vi "TDMS Main Page.vi"(8 "error in (no error)":errorcluster, 11 "Node Ptr":T2 format="%.0x") -> (0 "error out":errorcluster)   [LabVIEW 2011, in "TDMS Custom Device.lvlib"]
uses:
  TDMS Custom Device.lvlib
  <vilib>/NI Veristand/Custom Device API/Custom Device Item Ref.ctl
  <vilib>/NI Veristand/Custom Device API/Path Type.ctl
  <vilib>/NI Veristand/Custom Device API/Custom Device File Dependency.ctl
  <vilib>/NI Veristand/Custom Device API/Path Specification.ctl
  <vilib>/NI Veristand/Custom Device API/Custom Device Supported Target.ctl
  <vilib>/NI Veristand/Custom Device API/Set Item Property (Path).vi
  <vilib>/NI Veristand/Custom Device API/Custom Device API.lvlib
panel:
  out "# Samples":u32
  out "dt (sec)":dbl
  in  "Subheader":cluster{"Section Name":string}={"Section Name"="Buffering/Interpolation Default Settings"}
  in  "Fifo Depth":u32=200 min=1 max=400
  in  "Interpolation Width":i32=1 caption="The system uses this number of samples on either side of a point to be used by the above method. Increase to increase smoothness, decrease for performance." min=1 max=50
  in  "Interpolation Method":T1(ring)=enum."Linear"
  in  "View TDMS file":bool
  in  "Load Channels from File":bool
  in  "Header":cluster{"Section Name":string}={"Section Name"="TDMS Player Settings"}
  in  "Device Description (optional)":string
  in  "Name":string
  in  "Dependency":T4={"Source"={"TDMS Local Path"=path "", "Type"=enum."Absolute"}, "RT Path"=path "", "Force Download File?"=TRUE}
  # "Note: Used ONLY when 'Load Channels' is clicked."
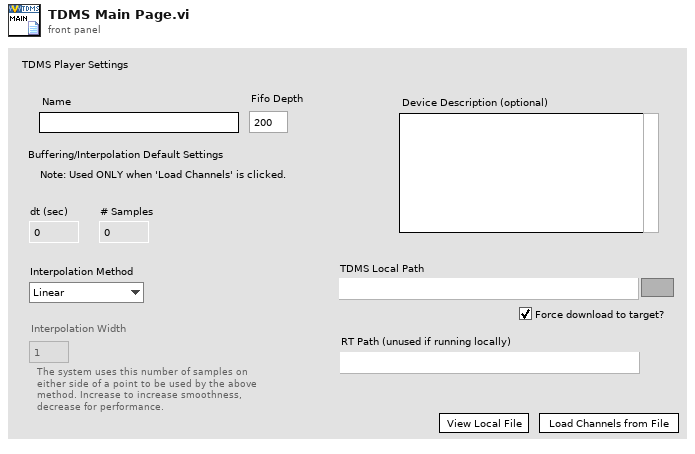
[diagram p1: front panel]
types:
  T1 = enum16{"Nearest", "Linear", "Spline", "Cubic Hermite", "Lagrange", "Polynomial"}
  T2 = typedef "Custom Device API.lvlib/Custom Device Item Ref.ctl" = u64
  T3 = typedef "Custom Device API.lvlib/Path Type.ctl" = enum16{"Absolute", "To Base", "To Common Data Dir", "To Application Data Dir"}
  T4 = cluster{"Source":cluster{"TDMS Local Path":path, "Type":T3}, "RT Path":path, "Force Download File?":bool}
  T5 = typedef "Custom Device API.lvlib/Custom Device Item Info.ctl" = cluster{"Name":string, "Is Channel":bool, "GUID":string}
  T6 = typedef "Custom Device API.lvlib/Custom Device File Dependency.ctl" = cluster{"Source":T7, "RT Destination":path, "ForceDownload?":bool, "SupportedTarget":T8, "Version":string}
  T7 = typedef "Custom Device API.lvlib/Path Specification.ctl" = cluster{"Path":path, "Type":T3}
  T8 = typedef "Custom Device API.lvlib/Custom Device Supported Target.ctl" = enum16{"All", "PharLap", "VxWorks", "Windows", "PharLap & Windows", "PharLap & VxWorks", "VxWorks & Windows"}
  T9 = typedef "Custom Device API.lvlib/Custom Device Channel.ctl" = cluster{"Type":T10, "Units":string, "Default Value":dbl, "Faultable":bool, "Scalable":bool}
  T10 = typedef "Custom Device API.lvlib/Custom Device Channel Type.ctl" = enum16{"Input", "Output"}
  T11 = enum8{"Enabled", "Disabled", "Disabled and Grayed Out"}
  T12 = typedef "Custom Device API.lvlib/Custom Device Commands.ctl" = enum16{"Default", "Item renamed", "Shutdown", "Dynamic button pressed"}
  T13 = cluster{bool, "dt (sec)":dbl, "Interpolation Method ":enum16{"Nearest", "Linear", "Spline", "Cubic Hermite", "Lagrange", "Polynomial"}, "Interpolation Width":i32}
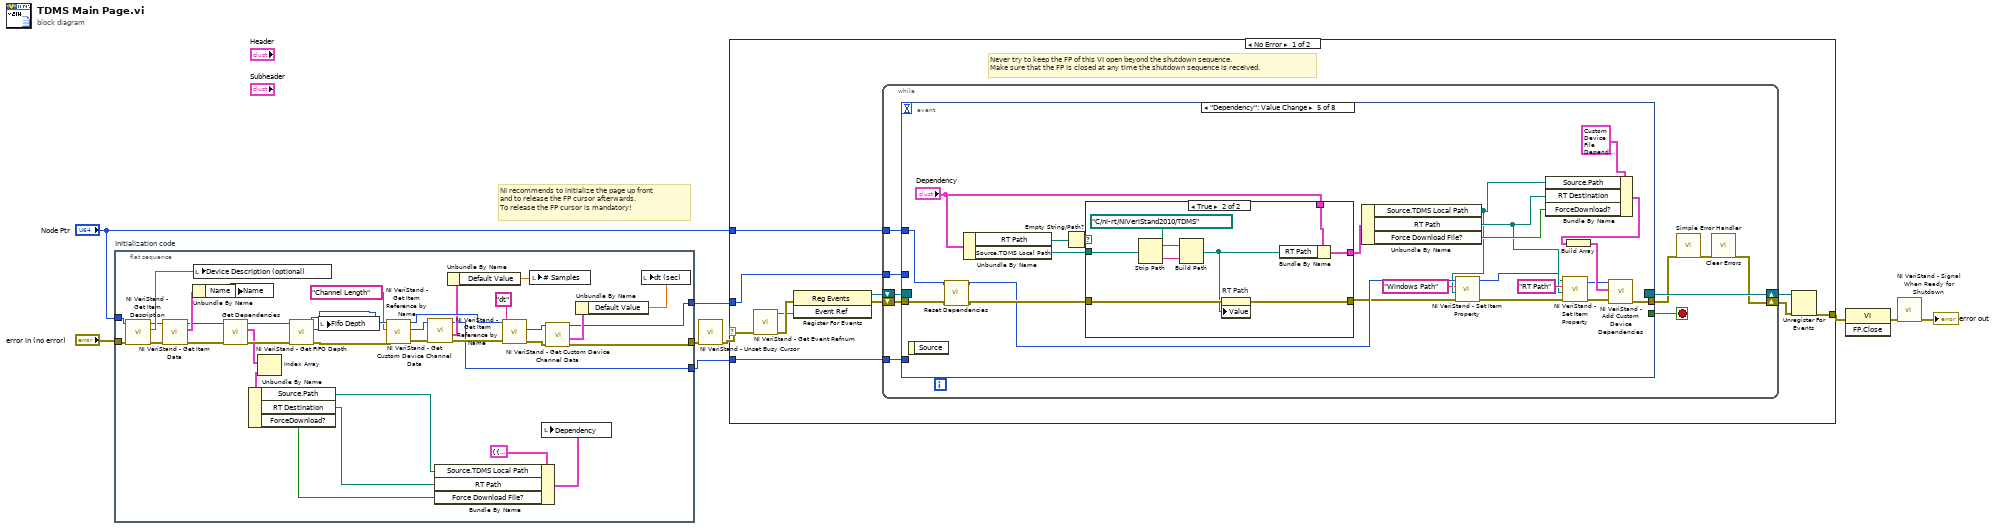
[diagram p0: block diagram]
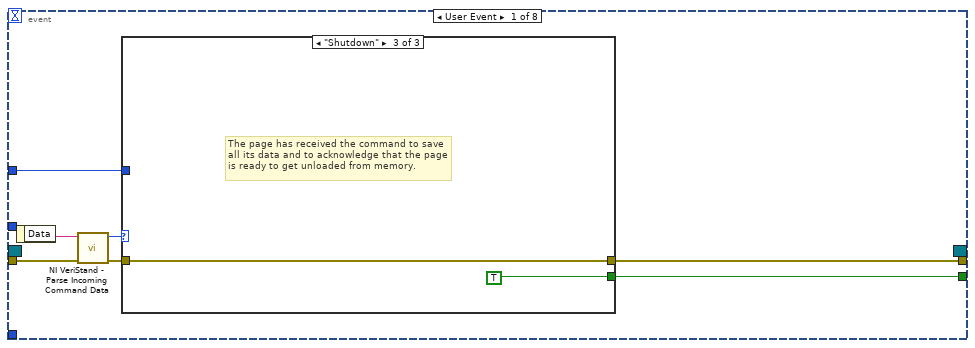
[diagram p2: hidden frame]
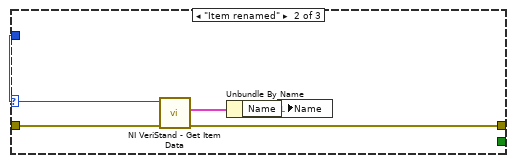
[diagram p4: hidden frame]
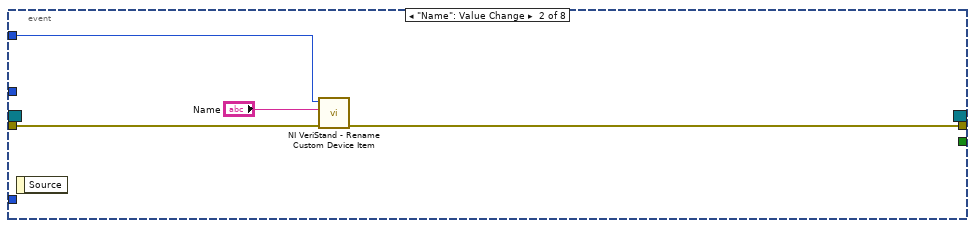
[diagram p5: hidden frame]
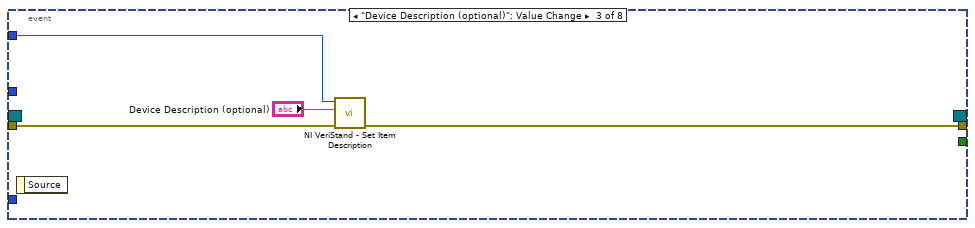
[diagram p6: hidden frame]
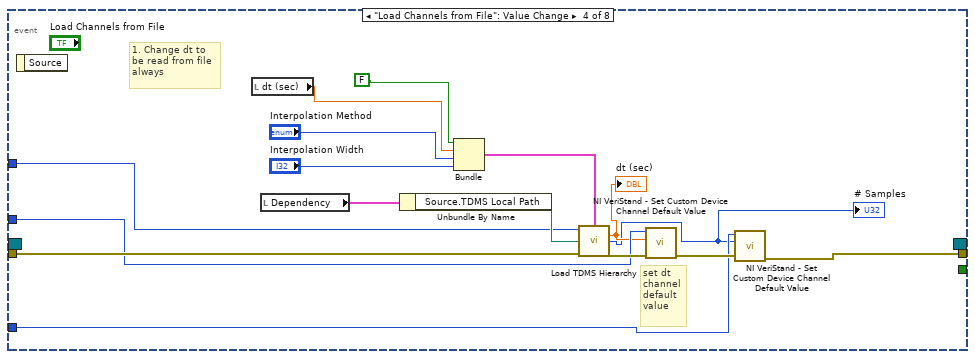
[diagram p7: hidden frame]
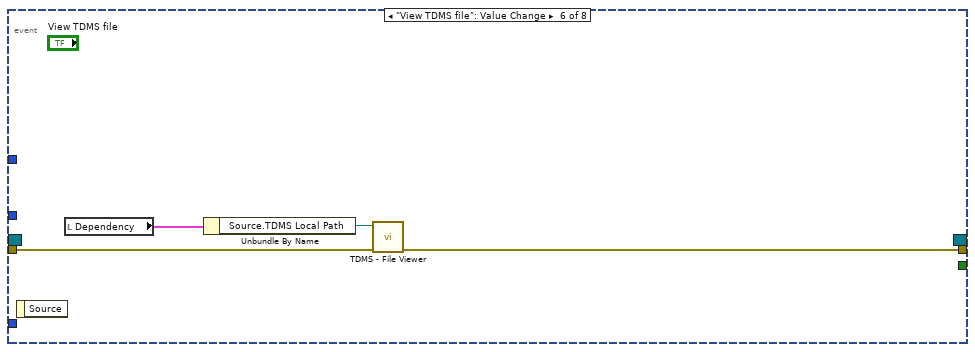
[diagram p9: hidden frame]
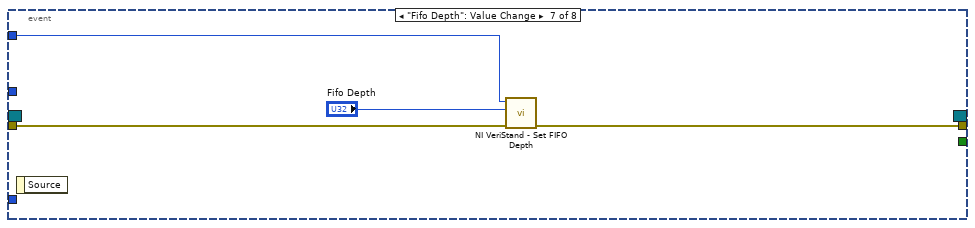
[diagram p10: hidden frame]
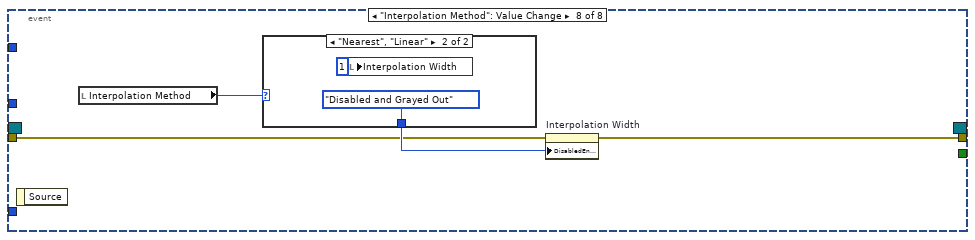
[diagram p11: hidden frame]
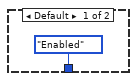
[diagram p12: hidden frame]
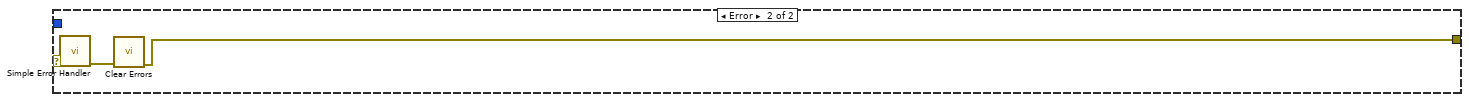
[diagram p13: hidden frame]
diagram:
  # "NI recommends to initialize the page up front\nand to release the FP cursor afterwards.\nTo release the FP cursor is mandatory!"
  n1 = flat-sequence "Initialization code" {
    tunnel: "error in (no error)" -> [w45]
    tunnel: "Node Ptr" -> [w44]
    tunnel: [w30] -> w5
    tunnel: [w27] -> w2
    tunnel: [w18] -> w1
    frame #0 {
      n2 = call <vilib>:"NI VeriStand - Get Item Description.vi"("error in (no error)"=w45, "Item Ref in"=w44) -> ("error out"=w42:errorcluster, "Description"=w43:string, "Item Ref out"=w41:T2)  [unwired: 7 out]
      n3 = call <vilib>:"NI VeriStand - Get Item Data.vi"("error in (no error)"=w42, "Item Ref in"=w41) -> ("error out"=w38:errorcluster, "Item Info"=w40:T5, "Item Ref out"=w37:T2)  [unwired: 7 out]
      n4 = Unbundle By Name(w40) -> ("Name"=w39:string)
      n5 = local write "Device Description (optional)"(w43) -> ()
      n6 = call "Get Dependencies.vi"("error in (no error)"=w38, "Device Ref in"=w37) -> ("error out"=w36:errorcluster, "Dependencies"=w11:T6[], "Dev Ref out"=w35:T2)  [unwired: 7 in]
      n7 = local write "Name"(w39) -> ()
      n8 = Index Array(array=w11) -> (element=w16:T6)  [unwired: 1 in]
      n9 = Unbundle By Name(w16) -> ("Source.Path"=w10:path, "RT Destination"=w14:path, "ForceDownload?"=w13:bool)
      n10 = call <vilib>:"NI VeriStand - Get FIFO Depth.vi"("error in (no error)"=w36, "Device Ref in"=w35) -> ("error out"=w26:errorcluster, "Size FIFO Source"=w34:u32, "Device Ref out"=w25:T2)  [unwired: 6 in, 1 out]
      n11 = local write "Fifo Depth"(w34) -> ()
      n12 = call <vilib>:"NI VeriStand - Get Item Reference by Name.vi"("error in (no error)"=w26, "Item Name"="Channel Length", "Parent Ref in"=w25) -> ("error out"=w21:errorcluster, "Item Ref"=w23:T2, "Parent Ref out"=w22:T2)  [unwired: 5 in, 1 out]
      n13 = call <vilib>:"NI VeriStand - Get Custom Device Channel Data.vi"("error in (no error)"=w21, "Channel Ref in"=w23) -> ("error out"=w19:errorcluster, "Channel"=w20:T9, "Channel Ref out"=w18:T2)  [unwired: 4 in, 3 out]
      n14 = Bundle By Name(cluster=T4 {"Source"={"TDMS Local Path"=path "", "Type"=enum."Absolute"}, "RT Path"=path "", "Force Download File?"=TRUE} ("Dependency"), "Source.TDMS Local Path"=w10, "RT Path"=w14, "Force Download File?"=w13) -> (w12:T4)
      n15 = Unbundle By Name(w20) -> ("Default Value"=w17:dbl)
      n16 = call <vilib>:"NI VeriStand - Get Item Reference by Name.vi"("error in (no error)"=w19, "Item Name"="dt", "Parent Ref in"=w22) -> ("error out"=w32:errorcluster, "Item Ref"=w31:T2)  [unwired: 5 in, 2 out]
      n17 = local write "# Samples"(w17) -> ()
      n18 = local write "Dependency"(w12) -> ()
      n19 = call <vilib>:"NI VeriStand - Get Custom Device Channel Data.vi"("error in (no error)"=w32, "Channel Ref in"=w31) -> ("error out"=w30:errorcluster, "Channel"=w29:T9, "Channel Ref out"=w27:T2)  [unwired: 4 in, 3 out]
      n20 = Unbundle By Name(w29) -> ("Default Value"=w28:dbl)
      n21 = local write "dt (sec)"(w28) -> ()
    }
  }
  n22 = call <vilib>:"NI VeriStand - Unset Busy Cursor.vi"("error in (no error)"=w5) -> ("error out"=w4:errorcluster)  [unwired: 10 out]
  n23 = case shown="No Error" w4 {
    selector: w4 -> [w48 w156]
    tunnel: [w53 w154] -> w9
    tunnel: "Node Ptr" -> [w49 _]
    tunnel: w2 -> [w47 _]
    tunnel: w1 -> [w46 _]
    frame No Error {
      # "Never try to keep the FP of this VI open beyond the shutdown sequence.\nMake sure that the FP is closed at any time the shutdown sequence is received."
      n24 = call <vilib>:"NI VeriStand - Get Event Refnum.vi"("error in (no error)"=w48) -> ("error out"=w56:errorcluster, "Event Ref"=w52:refnum<user-event>)  [unwired: 9 out]
      n25 = register-events(error in=w56, w52) -> (reference out=w50:refnum<event-registration>, error out=w51:errorcluster)  [unwired: 1 in]
      n26 = while {
        tunnel: w49 -> [w62]
        shift-right: [w59] -> w54
        shift-left: w51 -> [w65]
        shift-right: [w66] -> w55
        shift-left: w50 -> [w64]
        tunnel: w47 -> [w58]
        tunnel: w46 -> [w57]
        stop <- w63 stop-if-true
        n27 = event shown="[4] \"Dependency\": Value Change" {
          selector: w64 -> [_ _ _ _ _ _ _ _]
          dyn-events: [_ _ _ _ _ _ _ _] -> w66
          timeout: _ -> [_ _ _ _ _ _ _ _]
          tunnel: w65 -> [w73 w85 w88 w99 w121 w142 w145 w147]
          tunnel: [w69 _ _ _ _ _ _ _] -> w63
          tunnel: [w68 w84 w87 w91 w128 w141 w146 w149] -> w61
          tunnel: w62 -> [w67 w83 w89 w100 w120 _ w144 _]
          tunnel: w58 -> [_ _ _ w95 _ _ _ _]
          tunnel: w57 -> [_ _ _ w92 _ _ _ _]
          event User Event {
            n28 = event-data() -> ("Data"=w72:string)  [unwired: 1 out]
            n29 = call <vilib>:"NI VeriStand - Parse Incoming Command Data.vi"("error in (no error)"=w73, "Incoming data"=w72) -> ("error out"=w71:errorcluster, "Action"=w70:T12)  [unwired: 8 out]
            n30 = case shown="\"Shutdown\"" w70 {
              tunnel: w71 -> [w74 w79 w80]
              tunnel: [_ _ TRUE] -> w69
              tunnel: [w74 w76 w80] -> w68
              tunnel: w67 -> [_ w78 _]
              frame "Default", Default {
              }
              frame "Item renamed" {
                n31 = call <vilib>:"NI VeriStand - Get Item Data.vi"("error in (no error)"=w79, "Item Ref in"=w78) -> ("error out"=w76:errorcluster, "Item Info"=w77:T5)  [unwired: 8 out]
                n32 = Unbundle By Name(w77) -> ("Name"=w75:string)
                n33 = local write "Name"(w75) -> ()
              }
              frame "Shutdown" {
                # "The page has received the command to save all its data and to acknowledge that the page is ready to get unloaded from memory."
              }
            }
          }
          event "Name": Value Change {
            n34 = event-data() -> ()  [unwired: 2 out]
            n35 = call <vilib>:"NI VeriStand - Rename Custom Device Item.vi"("error in (no error)"=w85, "New Name"="Name", "Item Ref in"=w83) -> ("error out"=w84:errorcluster)  [unwired: 8 out]
          }
          event "Device Description (optional)": Value Change {
            n36 = event-data() -> ()  [unwired: 2 out]
            n37 = call <vilib>:"NI VeriStand - Set Item Description.vi"("error in (no error)"=w88, "Description"="Device Description (optional)", "Item Ref in"=w89) -> ("error out"=w87:errorcluster)  [unwired: 8 out]
          }
          event "Load Channels from File": Value Change {
            # "set dt \nchannel\ndefault \nvalue"
            # "1. Change dt to\nbe read from file\nalways"
            n38 = event-data() -> ()  [unwired: 2 out]
            n39 = local read "dt (sec)"() -> (w97:dbl)
            n40 = local read "Dependency"() -> (w101:T4)
            n41 = Unbundle By Name(w101) -> ("Source.TDMS Local Path"=w102:path)
            n42 = Bundle(FALSE, "dt (sec)"=w97, "Interpolation Method"="Interpolation Method", "Interpolation Width"="Interpolation Width") -> (w103:T13)  [unwired: 1 out]
            n43 = call "Load TDMS Hierarchy.vi"("Parent Ref in"=w100, "interpolation settings"=w103, "file path"=w102, "error in (no error)"=w99) -> ("dt out"=w94:dbl, "Samples"=w90:u32, "error out"=w96:errorcluster)  [unwired: 9 out]
            "dt (sec)" <- w94
            "# Samples" <- w90
            n44 = call <vilib>:"NI VeriStand - Set Custom Device Channel Default Value.vi"("error in (no error)"=w96, "Default Value"=w94, "Channel Ref in"=w95) -> ("error out"=w93:errorcluster)  [unwired: 7 in, 1 out]
            n45 = call <vilib>:"NI VeriStand - Set Custom Device Channel Default Value.vi"("error in (no error)"=w93, "Default Value"=w90, "Channel Ref in"=w92) -> ("error out"=w91:errorcluster)  [unwired: 7 in, 1 out]
          }
          event "Dependency": Value Change {
            n46 = event-data() -> ()  [unwired: 2 out]
            n47 = call "Reset Dependencies.vi"("error in (no error)"=w121, "Device Ref in"=w120) -> ("error out"=w122:errorcluster, "Dev Ref out"=w111:T2)  [unwired: 8 in]
            n48 = Unbundle By Name("Dependency") -> ("RT Path"=w126:path, "Source.TDMS Local Path"=w125:path)
            n49 = Empty String/Path?(string/path=w126) -> (empty?=w127:bool)
            n50 = case shown="True" w127 {
              tunnel: "Dependency" -> [w130 w136]
              tunnel: [w130 w135] -> w118
              tunnel: w122 -> [w129 w133]
              tunnel: [w129 w134] -> w110
              tunnel: w125 -> [_ w131]
              frame False {
                # "Use the already specified path"
              }
              frame True {
                n51 = Strip Path(path=w131) -> (name=w137:string)  [unwired: 1 out]
                n52 = Build Path(base path=path "C:/ni-rt/NIVeriStand2010/TDMS", name or relative path=w137) -> (appended path=w132:path)
                n53 = property on="RT Path" class="Path"(error in=w133, "Value"=w132) -> (error out=w134:errorcluster)  [unwired: 1 in, 1 out]
                n54 = Bundle By Name(cluster=w136, "RT Path"=w132) -> (w135:T4)
              }
            }
            n55 = Unbundle By Name(w118) -> ("Source.TDMS Local Path"=w107:path, "RT Path"=w112:path, "Force Download File?"=w124:bool)
            n56 = call-poly <vilib>:"NI VeriStand - Set Item Property.vi"("error in (no error)"=w110, "Value"=w107, "Property Name"="Windows Path", "Item Ref in"=w111) -> ("error out"=w109:errorcluster, "Item Ref out"=w108:T2)  [unwired: 5 in, 1 out]
            n57 = Bundle By Name(cluster=T6 {"Source"={"Path"=path "", "Type"=enum."Absolute"}, "RT Destination"=path "", "ForceDownload?"=FALSE, "SupportedTarget"=enum."PharLap", "Version"=""} ("Dependency"), "Source.Path"=w107, "RT Destination"=w112, "ForceDownload?"=w124) -> (w117:T6)
            n58 = call-poly <vilib>:"NI VeriStand - Set Item Property.vi"("error in (no error)"=w109, "Value"=w112, "Property Name"="RT Path", "Item Ref in"=w108) -> ("error out"=w115:errorcluster, "Item Ref out"=w114:T2)  [unwired: 5 in, 1 out]
            n59 = Build Array(w117) -> (w116:T6[])
            n60 = call <vilib>:"NI VeriStand - Add Custom Device Dependencies.vi"("error in (no error)"=w115, "Dependencies"=w116, "Device Ref in"=w114) -> ("error out"=w128:errorcluster)  [unwired: 8 out]
          }
          event "View TDMS file": Value Change {
            n61 = event-data() -> ()  [unwired: 2 out]
            n62 = local read "Dependency"() -> (w140:T4)
            n63 = Unbundle By Name(w140) -> ("Source.TDMS Local Path"=w139:path)
            n64 = call <vilib>:"TDMS - File Viewer.vi"("error in (no error)"=w142, "file path"=w139) -> ("error out"=w141:errorcluster)  [unwired: 5 out]
          }
          event "Fifo Depth": Value Change {
            n65 = event-data() -> ()  [unwired: 2 out]
            n66 = call <vilib>:"NI VeriStand - Set FIFO Depth.vi"("error in (no error)"=w145, "Size FIFO Source (1)"="Fifo Depth", "Device Ref in"=w144) -> ("error out"=w146:errorcluster)  [unwired: 7 in, 1 out]
          }
          event "Interpolation Method": Value Change {
            n67 = event-data() -> ()  [unwired: 2 out]
            n68 = local read "Interpolation Method"() -> (w150:T1)
            n69 = case shown="\"Nearest\", \"Linear\"" w150 {
              tunnel: [T11."Enabled" ("Disabled") T11."Disabled and Grayed Out" ("Disabled")] -> w148
              frame Default {
              }
              frame "Nearest", "Linear" {
                n70 = local write "Interpolation Width"(1 ("Interpolation Width")) -> ()
              }
            }
            n71 = property on="Interpolation Width" class="DigNum (strict)"(error in=w147, "DisabledEnum"=w148) -> (error out=w149:errorcluster)  [unwired: 1 in, 1 out]
          }
        }
        n72 = call <vilib>:"Simple Error Handler.vi"("error in (no error)"=w61) -> ("error out"=w60:errorcluster)  [unwired: 1 in, 7 out]
        n73 = call <vilib>:"Clear Errors.vi"("error in (no error)"=w60) -> ("error out"=w59:errorcluster)  [unwired: 6 out]
      }
      n74 = Unregister For Events(event registration refnum=w55, error in=w54) -> (error out=w53:errorcluster)
    }
    frame Error {
      n75 = call <vilib>:"Simple Error Handler.vi"("error in (no error)"=w156) -> ("error out"=w155:errorcluster)  [unwired: 1 in, 7 out]
      n76 = call <vilib>:"Clear Errors.vi"("error in (no error)"=w155) -> ("error out"=w154:errorcluster)  [unwired: 6 out]
    }
  }
  n77 = invoke class="VI" method="FP.Close"(error in=w9) -> (error out=w8:errorcluster)  [unwired: 2 in, 2 out]
  n78 = call <vilib>:"NI VeriStand - Signal When Ready for Shutdown.vi"("error in (no error)"=w8) -> ("error out"=→"error out":errorcluster)  [unwired: 10 out]
